vi "Tester.vi"() -> ()   [LabVIEW 2016]
uses:
  Mover/Mover.lvclass
  PVector.lvclass
  Forces/Friction/Friction.lvclass
panel:
  out "Mover out":refnum<class "Mover.lvclass">
  out "Y 3":dbl
  out "X 3":dbl
  out "Mag(V) 3":dbl
  out "Angle 3":dbl
  out "Y 2":dbl
  out "X 2":dbl
  out "Angle 2":dbl
  out "Mag(V) 2":dbl
  out "Angle":dbl
  out "Mag(norm(V))":dbl
  out "Mag(V)":dbl
  in  "Y":dbl
  in  "X":dbl
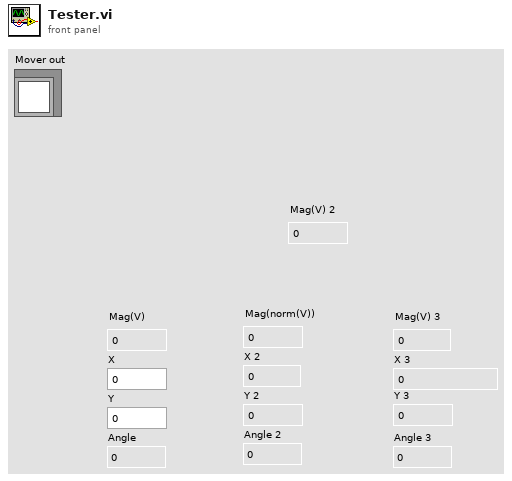
[diagram p1: front panel]
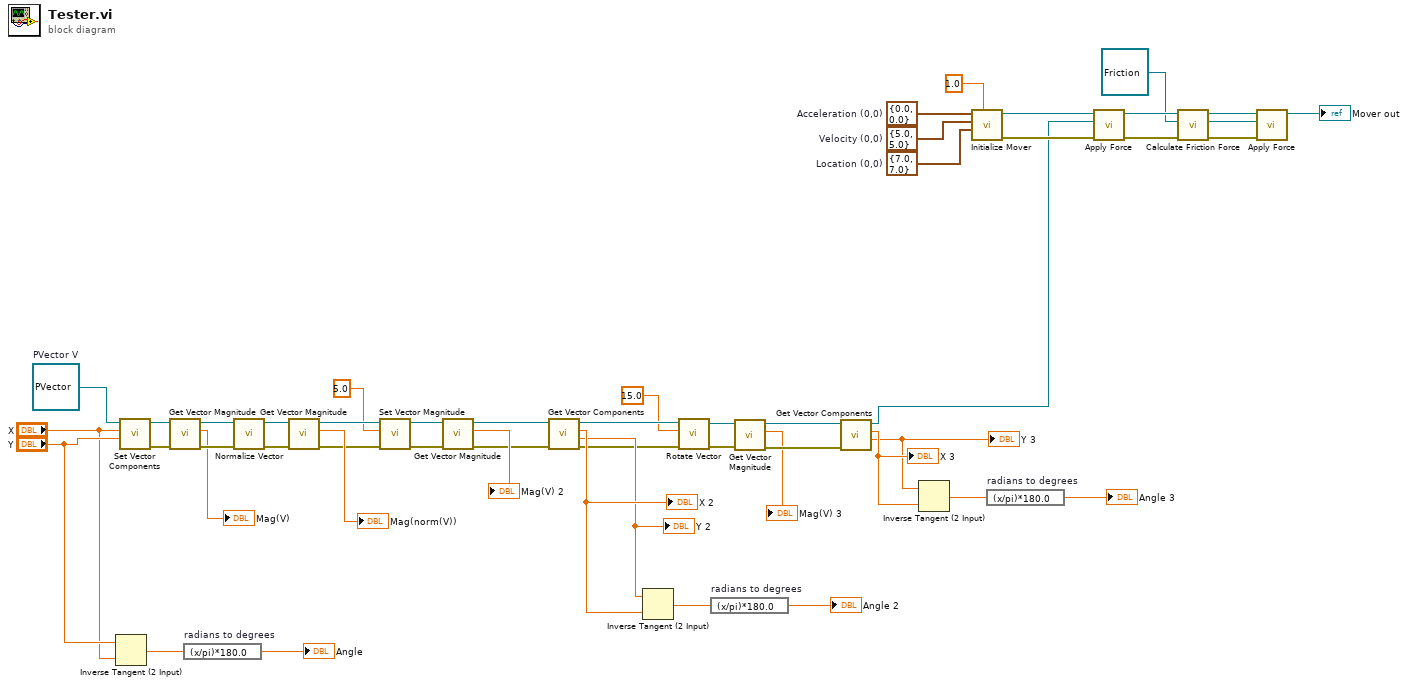
[diagram p0: block diagram]
diagram:
  w10 = cluster{"X":dbl, "Y":dbl} {"X"=7.0, "Y"=7.0}  # Location (0,0)
  w11 = cluster{"X":dbl, "Y":dbl} {"X"=5.0, "Y"=5.0}  # Velocity (0,0)
  w12 = cluster{"X":dbl, "Y":dbl} {"X"=0.0, "Y"=0.0}  # Acceleration (0,0)
  w51 = refnum<class "PVector.lvclass"> refnum  # PVector V
  n1 = Inverse Tangent (2 Input)(1:"X", 2:"Y") -> (0:w40:dbl)
  n2 = call "Set Vector Components.vi"("Y"="Y", "X"="X", "PVector in"=w51) -> ("error out"=w48:errorcluster, "PVector out"=w50:refnum<class "PVector.lvclass">)  [unwired: 7 in]
  n3 = call "Get Vector Magnitude.vi"("error in"=w48, "PVector in"=w50) -> ("error out"=w47:errorcluster, "Mag(V)"=→"Mag(V)":dbl, "PVector out"=w49:refnum<class "PVector.lvclass">)  [unwired: 7 in]
  n4 = expression code="(x/pi)*180.0" "radians to degrees"(w40) -> (→"Angle":dbl)
  n5 = call "Normalize Vector.vi"("error in"=w47, "PVector in"=w49) -> ("error out"=w45:errorcluster, "norm(PVector) out"=w46:refnum<class "PVector.lvclass">)  [unwired: 8 in]
  n6 = call "Get Vector Magnitude.vi"("error in"=w45, "PVector in"=w46) -> ("error out"=w38:errorcluster, "Mag(V)"=→"Mag(norm(V))":dbl, "PVector out"=w37:refnum<class "PVector.lvclass">)  [unwired: 7 in]
  n7 = call "Set Vector Magnitude.vi"("error in"=w38, "Manitude"=5.0, "PVector in"=w37) -> ("error out"=w35:errorcluster, "PVector out"=w34:refnum<class "PVector.lvclass">)  [unwired: 7 in]
  n8 = call "Get Vector Magnitude.vi"("error in"=w35, "PVector in"=w34) -> ("error out"=w32:errorcluster, "Mag(V)"=→"Mag(V) 2":dbl, "PVector out"=w31:refnum<class "PVector.lvclass">)  [unwired: 7 in]
  n9 = call "Get Vector Components.vi"("error in"=w32, "PVector in"=w31) -> ("error out"=w26:errorcluster, "Y"=w27:dbl, "X"=w28:dbl, "PVector out"=w25:refnum<class "PVector.lvclass">)  [unwired: 6 in]
  "X 2" <- w28
  "Y 2" <- w27
  n10 = Inverse Tangent (2 Input)(1:w28, 2:w27) -> (0:w30:dbl)
  n11 = call "Rotate Vector.vi"("error in"=w26, "Angle [180,-180]"=15.0, "PVector in"=w25) -> ("error out"=w22:errorcluster, "PVector out"=w21:refnum<class "PVector.lvclass">)  [unwired: 7 in]
  n12 = expression code="(x/pi)*180.0" "radians to degrees"(w30) -> (→"Angle 2":dbl)
  n13 = call "Get Vector Magnitude.vi"("error in"=w22, "PVector in"=w21) -> ("error out"=w24:errorcluster, "Mag(V)"=→"Mag(V) 3":dbl, "PVector out"=w23:refnum<class "PVector.lvclass">)  [unwired: 7 in]
  n14 = call "Get Vector Components.vi"("error in"=w24, "PVector in"=w23) -> ("Y"=w16:dbl, "X"=w17:dbl, "PVector out"=w8:refnum<class "PVector.lvclass">)  [unwired: 6 in, 1 out]
  "X 3" <- w17
  "Y 3" <- w16
  n15 = Inverse Tangent (2 Input)(1:w17, 2:w16) -> (0:w20:dbl)
  n16 = call "Initialize Mover.vi"("Mass (1)"=1.0, "Location (0,0)"=w10, "Velocity (0,0)"=w11, "Acceleration (0,0)"=w12) -> ("error out"=w9:errorcluster, "Mover out"=w14:refnum<class "Mover.lvclass">)  [unwired: 6 in]
  n17 = expression code="(x/pi)*180.0" "radians to degrees"(w20) -> (→"Angle 3":dbl)
  n18 = call "Apply Force.vi"("error in"=w9, "Force Vector"=w8, "Mover in"=w14) -> ("error out"=w6:errorcluster, "Mover out"=w7:refnum<class "Mover.lvclass">)  [unwired: 7 in]
  n19 = call "Calculate Friction Force.vi"("error in"=w6, "Friction in"=refnum<class "Friction.lvclass"> refnum, "Mover in"=w7) -> ("error out"=w5:errorcluster, "Friction Force out"=w3:refnum<class "PVector.lvclass">, "Mover out"=w4:refnum<class "Mover.lvclass">)  [unwired: 6 in]
  n20 = call "Apply Force.vi"("error in"=w5, "Force Vector"=w3, "Mover in"=w4) -> ("Mover out"=→"Mover out":refnum<class "Mover.lvclass">)  [unwired: 7 in, 1 out]
